vi "Get Range Averages.vi"(10 "Upper Bounds":dbl[](array[numeric]), 11 "Lower Bounds":dbl[](array[numeric])) -> (3 "Array":dbl[](array[numeric]))   [LabVIEW 2012]
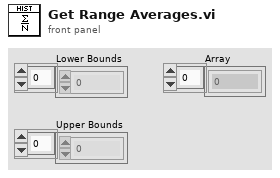
[diagram p1: front panel]
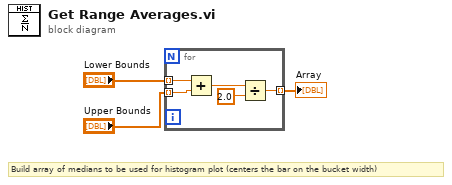
[diagram p0: block diagram]
diagram:
  # "Build array of medians to be used for histogram plot (centers the bar on the bucket width)"
  n1 = for {
    tunnel: "Lower Bounds" -> [w8] mode=indexing
    tunnel: "Upper Bounds" -> [w7] mode=indexing
    tunnel: [w4] -> w3 mode=indexing
    n2 = Add(x=w8, y=w7) -> (x+y=w6:dbl)
    n3 = Divide(x=w6, y=2.0) -> (x/y=w4:dbl)
  }
  "Array" <- w3
